vi "FGV_Init.vi"(8 "error in":errorcluster) -> (0 "error out":errorcluster)   [LabVIEW 2026]
uses:
  TypeDef_FGV.ctl
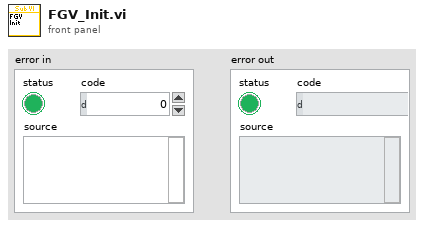
[diagram p1: front panel]
types:
  T1 = typedef "TypeDef_FGV.ctl" = enum16{"Initialize", "Write", "Read", "Read_File", "Write_to_File"}
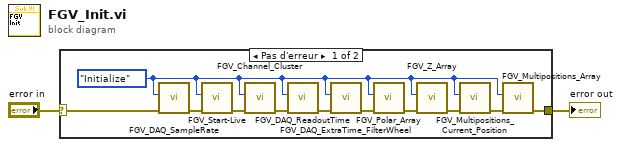
[diagram p0: block diagram]
diagram:
  n1 = case shown="Pas d'erreur" "error in" {
    selector: "error in" -> [w4 w14]
    tunnel: [w3 w14] -> w1
    frame No Error {
      w6 = TypeDef_FGV."Initialize" ("Action")
      n2 = call "FGV_DAQ_SampleRate.vi"("error in"=w4, "Action"=w6) -> ("error out"=w13:errorcluster)  [unwired: 8 in, 1 out]
      n3 = call "FGV_Start-Live.vi"("error in"=w13, "Action"=w6) -> ("error out"=w12:errorcluster)  [unwired: 8 in, 1 out]
      n4 = call "FGV_Channel_Cluster.vi"("error in"=w12, "Action"=w6) -> ("error out"=w11:errorcluster)  [unwired: 8 in, 1 out]
      n5 = call "FGV_DAQ_ReadoutTime.vi"("error in"=w11, "Action"=w6) -> ("error out"=w10:errorcluster)  [unwired: 8 in, 1 out]
      n6 = call "FGV_DAQ_ExtraTime_FilterWheel.vi"("error in"=w10, "Action"=w6) -> ("error out"=w9:errorcluster)  [unwired: 8 in, 1 out]
      n7 = call "FGV_Polar_Array.vi"("error in"=w9, "Action"=w6) -> ("error out"=w8:errorcluster)  [unwired: 7 in, 2 out]
      n8 = call "FGV_Z_Array.vi"("error in"=w8, "Action"=w6) -> ("error out"=w7:errorcluster)  [unwired: 7 in, 2 out]
      n9 = call "FGV_Multipositions_Current_Position.vi"("error in"=w7, "Action"=w6) -> ("error out"=w5:errorcluster)  [unwired: 8 in, 1 out]
      n10 = call "FGV_Multipositions_Array.vi"("error in"=w5, "Action"=w6) -> ("error out"=w3:errorcluster)  [unwired: 7 in, 2 out]
    }
    frame Error {
    }
  }
  "error out" <- w1
